vi "20211015_07.vi"() -> ()   [LabVIEW 2019]
panel:
  out "Time":timestamp format="%<%x %.3X>T"
  out "Clock":T1(knob)={"Numeric"=0.0, "Numeric"=0.0, "Numeric"=6.0} scale=0.0..12.0
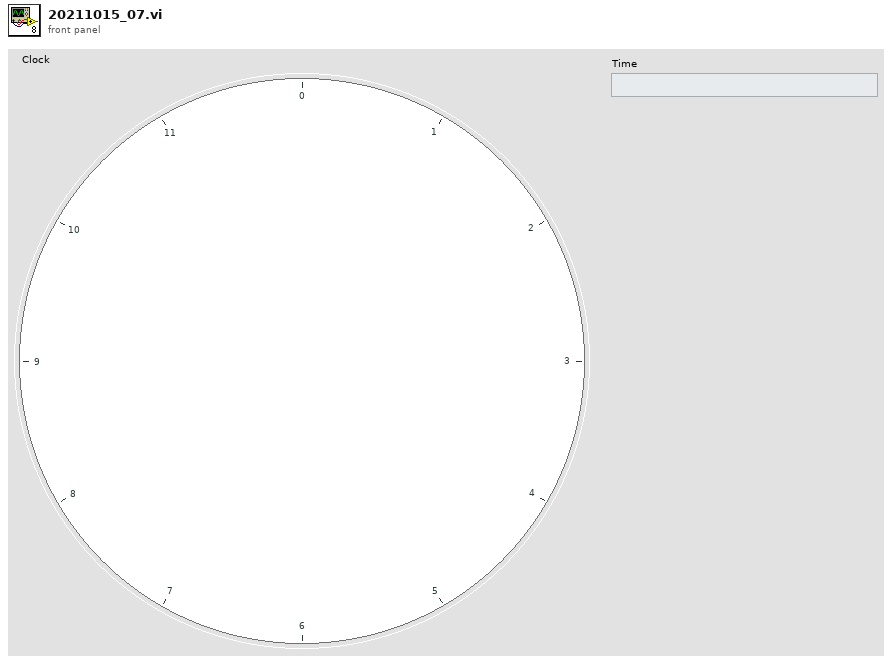
[diagram p1: front panel]
types:
  T1 = cluster{"Numeric":dbl, "Numeric":dbl, "Numeric":dbl}
  T2 = typedef "LVDateTimeRec.ctl" = cluster{"fractional second":dbl, "second":i32, "minute":i32, "hour":i32, "day of month":i32, "month":i32, "year":i32, "day of week":i32, "day of year":i32, "DST":i32}
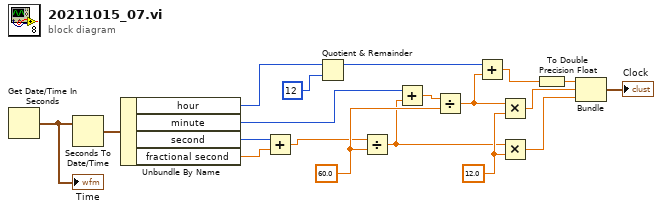
[diagram p0: block diagram]
diagram:
  w16 = 12.0 ("y")
  w17 = 60.0 ("y")
  n1 = Get Date/Time In Seconds() -> (seconds since 1Jan1904=w12:timestamp)
  "Time" <- w12
  n2 = Seconds To Date/Time(time stamp (now)=w12) -> (date time rec=w19:T2)  [unwired: 1 in]
  n3 = Unbundle By Name(w19) -> ("hour"=w9:i32, "minute"=w6:i32, "second"=w7:i32, "fractional second"=w11:dbl)
  n4 = Add(x=w7, y=w11) -> (x+y=w10:dbl)
  n5 = Quotient & Remainder(x=w9, y=12) -> (x-y*floor(x/y)=w4:i32)  [unwired: 1 out]
  n6 = Divide(x=w10, y=w17) -> (x/y=w5:dbl)
  n7 = Add(x=w6, y=w5) -> (x+y=w3:dbl)
  n8 = Divide(x=w3, y=w17) -> (x/y=w1:dbl)
  n9 = Add(x=w4, y=w1) -> (x+y=w2:dbl)
  n10 = Multiply(x=w1, y=w16) -> (x*y=w15:dbl)
  n11 = Multiply(x=w5, y=w16) -> (x*y=w14:dbl)
  n12 = To Double Precision Float(number=w2) -> (double precision float=w13:dbl)
  n13 = Bundle(w13, w15, w14) -> (→"Clock":cluster{dbl, dbl, dbl})  [unwired: 1 in]
